vi "短日期时间转长日期格式.vi"(11 "data":string[][](table)) -> (3 "输出数组":string[][](array[string]))   [LabVIEW 2016]
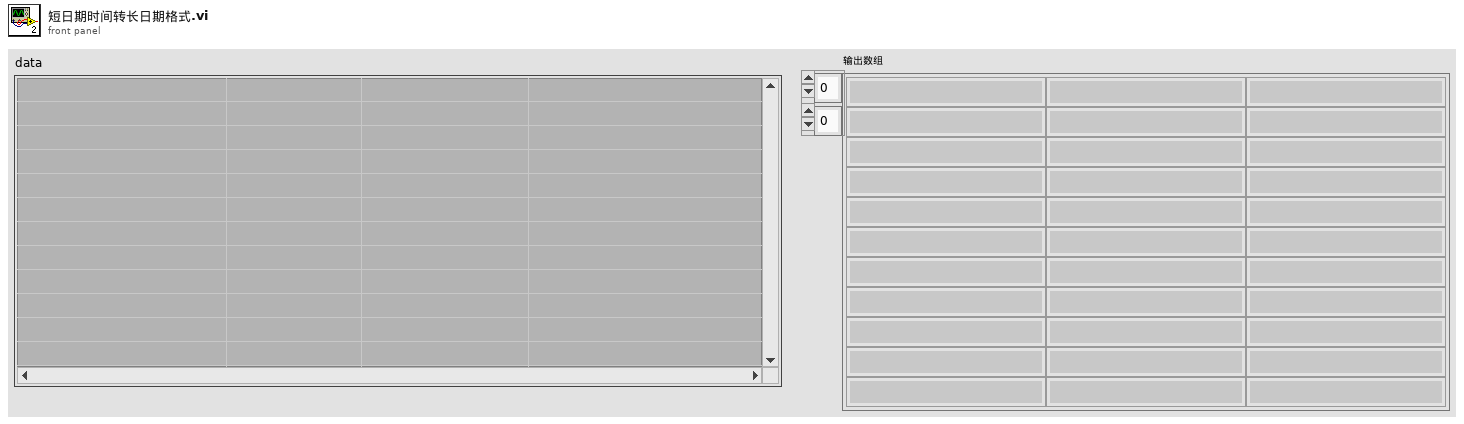
[diagram p1: front panel]
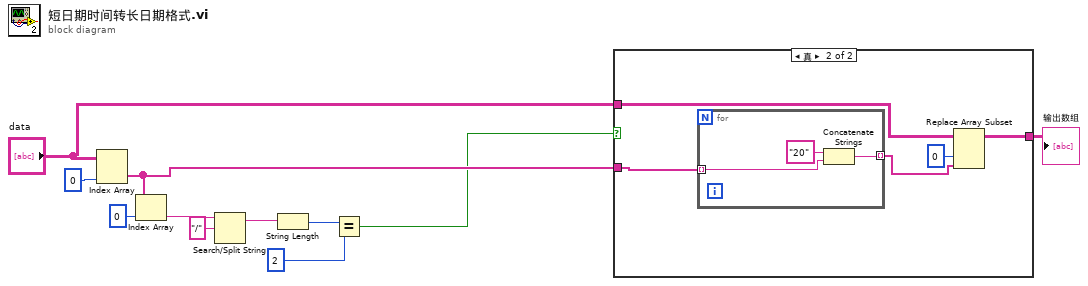
[diagram p0: block diagram]
diagram:
  n1 = Index Array(array="data", index (col)=0 ("禁用的索引 (列)")) -> (element=w8:string[])  [unwired: 1 in]
  n2 = Index Array(array=w8, index=0 ("索引")) -> (element=w6:string)
  n3 = Search/Split String(string=w6, search string/char (-)="/" ("搜索字符串/字符(-)")) -> (substring before match=w4:string)  [unwired: 1 in, 2 out]
  n4 = String Length(string=w4) -> (length=w3:i32)
  n5 = Equal?(x=w3, y=2) -> (x = y?=w1:bool)
  n6 = case shown="真" w1 {
    tunnel: w8 -> [_ w17]
    tunnel: "data" -> [w12 w16]
    tunnel: [w12 w13] -> w9
    frame False {
    }
    frame True {
      n7 = for {
        tunnel: w17 -> [w20] mode=indexing
        tunnel: [w18] -> w14 mode=indexing
        n8 = Concatenate Strings("20" ("字符串"), w20) -> (w18:string)
      }
      n9 = Replace Array Subset(array=w16, new element=w14, index (col)=0 ("禁用的索引 (列)")) -> (w13:string[][])  [unwired: 1 in]
    }
  }
  "输出数组" <- w9
